vi "FGV ALL REFS.vi"(0 "name":string, 2 "Ctl Refnum in":refnum<vi>, 12 "CMD":T1) -> (20 "Ctl Refnum out":refnum<vi>)   [LabVIEW 2020]
uses:
  PCT FGV CMD.ctl
panel:
  out "error out":errorcluster
  in  "error in (no error)":errorcluster
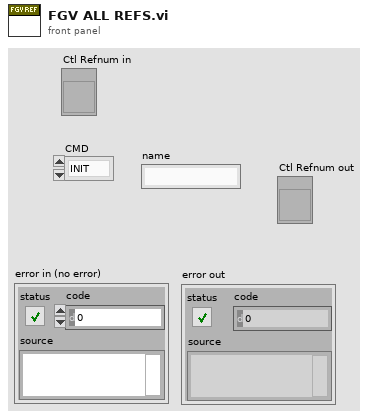
[diagram p1: front panel]
types:
  T1 = typedef "PCT FGV CMD.ctl" = enum16{"INIT", "GET", "SET"}
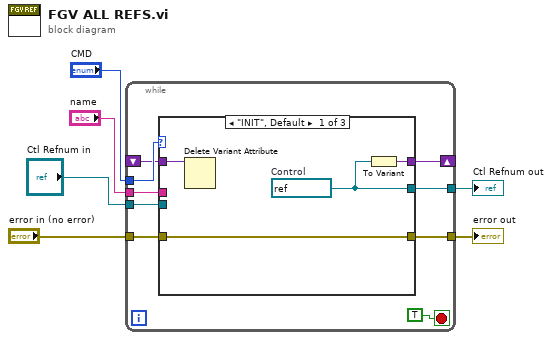
[diagram p0: block diagram]
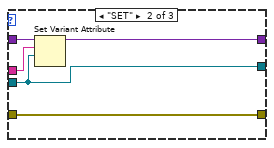
[diagram p2: hidden frame]
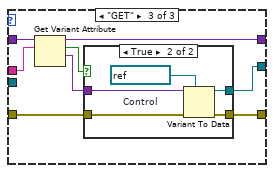
[diagram p3: hidden frame]
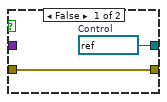
[diagram p4: hidden frame]
diagram:
  n1 = while {
    tunnel: "CMD" -> [w14]
    shift-right: [w13] -> _
    shift-left: _ -> [w12]
    tunnel: "name" -> [w11]
    tunnel: [w10] -> w4
    tunnel: [w9] -> w3
    tunnel: "error in (no error)" -> [w8]
    tunnel: "Ctl Refnum in" -> [w7]
    stop <- TRUE stop-if-true
    n2 = case shown="\"INIT\", Default" w14 {
      tunnel: [w16 w22 w28] -> w13
      tunnel: w12 -> [w19 w23 w32]
      tunnel: w11 -> [_ w21 w31]
      tunnel: [w17 w20 w29] -> w10
      tunnel: [w18 w24 w25] -> w9
      tunnel: w8 -> [w18 w24 w26]
      tunnel: w7 -> [_ w20 _]
      frame "INIT", Default {
        w17 = refnum<vi> refnum  # Control
        n3 = Delete Variant Attribute(7:w19) -> ()  [unwired: 2 in, 3 out]
        n4 = To Variant(anything=w17) -> (Variant=w16:variant)
      }
      frame "SET" {
        n5 = Set Variant Attribute(Variant=w23, name=w21, value=w20) -> (Variant out=w22:variant)  [unwired: 1 in, 2 out]
      }
      frame "GET" {
        n6 = Get Variant Attribute(Variant=w32, name=w31) -> (duplicate Variant=w28:variant, found=w27:bool, value=w30:variant)  [unwired: 2 in, 1 out]
        n7 = case shown="True" w27 {
          tunnel: w30 -> [_ w39]
          tunnel: [w33 w37] -> w29
          tunnel: w26 -> [w34 w36]
          tunnel: [w34 w35] -> w25
          frame False {
            w33 = refnum<vi> refnum  # Control
          }
          frame True {
            w38 = refnum<vi> refnum  # Control
            n8 = Variant To Data(error in=w36, type=w38, Variant=w39) -> (data=w37:refnum<vi>, error out=w35:errorcluster)
          }
        }
      }
    }
  }
  "error out" <- w3
  "Ctl Refnum out" <- w4
